vi "robotimageprocessing2.vi"(0 "Image In":T2, 7 "error in":errorcluster) -> (20 "Image Out":T2, 21 "Number of Matches (Shape Matching 1)":i32, 22 "Shape Report (Shape Matching 1)":T1(array[cluster]) {"Score" format="%.2f"; "Centroid"."y" format="%.2f"; "Centroid"."x" format="%.2f"}, 23 "Shape Report (calibrated) (Shape Matching 1)":T1(array[cluster]) {"Score" format="%.2f"; "Centroid"."y" format="%.2f"; "Centroid"."x" format="%.2f"}, 27 "error out":errorcluster)   [LabVIEW 2015]
uses:
  <vilib>/vision/Image Controls.llb/IMAQ Image.ctl
  <vilib>/vision/NI_Vision_Development_Module.lvlib
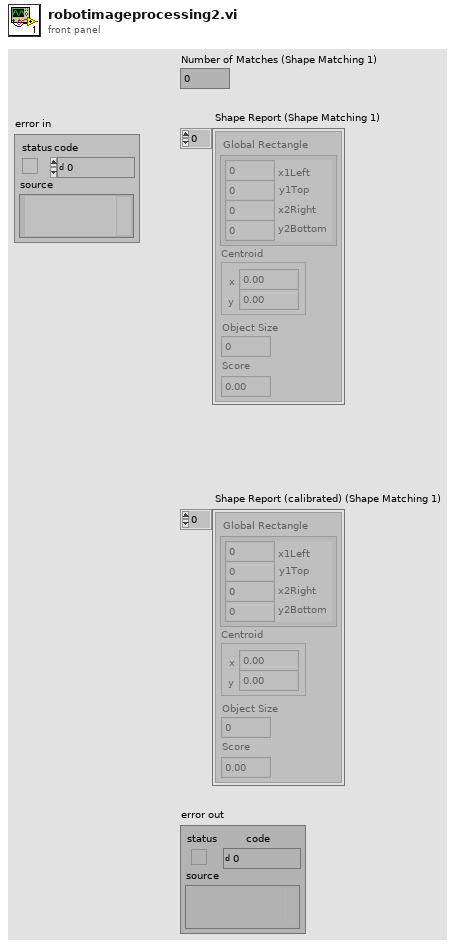
[diagram p1: front panel]
types:
  T1 = cluster{"Global Rectangle":cluster{"x1Left":i32, "y1Top":i32, "x2Right":i32, "y2Bottom":i32}, "Centroid":cluster{"x":sgl, "y":sgl}, "Object Size":u32, "Score":dbl}[]
  T2 = typedef "IMAQ Image.ctl" = refnum<image>
  T3 = enum32{"AutoM", "Close", "Dilate", "Erode", "Gradient", "Gradient out", "Gradient in", "Hit miss", "Open", "PClose", "POpen", "Thick", "Thin"}
  T4 = cluster{"Measurement Parameter":i32, "Range Lower Value":dbl, "Range Upper Value":dbl, "Range":bool, "Measurement Type":bool}[]
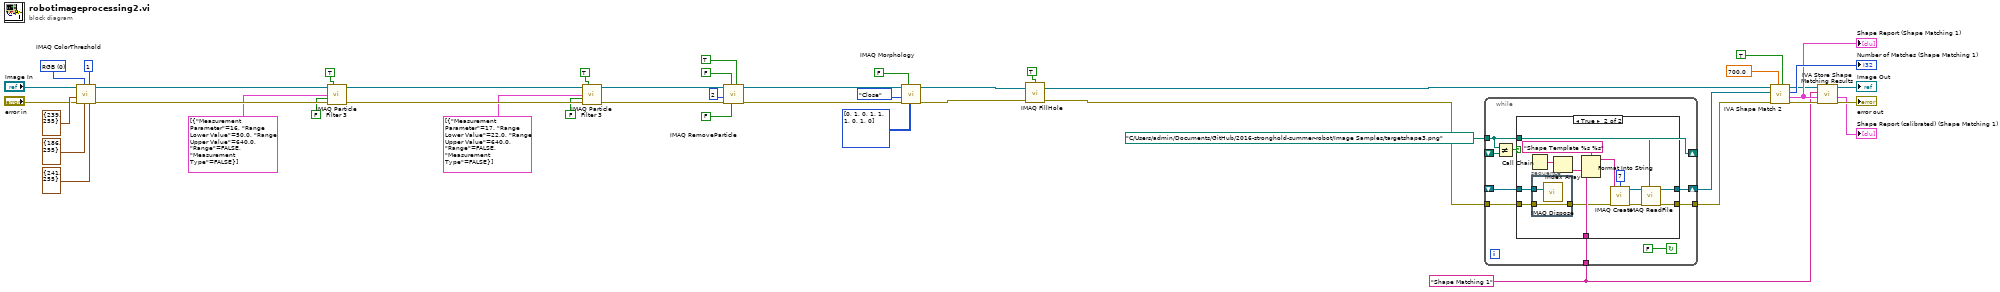
[diagram p0: block diagram]
diagram:
  w1 = "Shape Matching 1" ("Step Name")
  w45 = u16 0 items=["RGB", "HSL", "HSV", "HSI"] ("Color Mode")
  n1 = call "IMAQ ColorThreshold"("Blue or Luma or Val or Inten Range"=cluster{"Lower value":i32, "Upper value":i32} {"Lower value"=241, "Upper value"=255}, "Replace Value"=1, "Green or Sat Range"=cluster{"Lower value":i32, "Upper value":i32} {"Lower value"=186, "Upper value"=255}, "Color Mode"=w45, "error in (no error)"="error in", "Red or Hue Range"=cluster{"Lower value":i32, "Upper value":i32} {"Lower value"=239, "Upper value"=255}, "Image Src"="Image In") -> ("error out"=w39:errorcluster, "Image Dst Out"=w35:T2)  [unwired: 1 in, 2 out]
  n2 = call "IMAQ Particle Filter 3"("Image Src"=w35, "Connectivity 4/8 (8)"=TRUE, "Selection Values"=T4 [{"Measurement Parameter"=16, "Range Lower Value"=50.0, "Range Upper Value"=640.0, "Range"=FALSE, "Measurement Type"=FALSE}], "Keep/Remove Particles (F)"=FALSE ("Keep/Remove Particles"), "error in (no error)"=w39) -> ("Image Dst Out"=w30:T2, "error out"=w36:errorcluster)  [unwired: 4 in, 5 out]
  n3 = call "IMAQ Particle Filter 3"("Image Src"=w30, "Connectivity 4/8 (8)"=TRUE, "Selection Values"=T4 [{"Measurement Parameter"=17, "Range Lower Value"=22.0, "Range Upper Value"=640.0, "Range"=FALSE, "Measurement Type"=FALSE}], "Keep/Remove Particles (F)"=FALSE ("Keep/Remove Particles"), "error in (no error)"=w36) -> ("Image Dst Out"=w24:T2, "error out"=w31:errorcluster)  [unwired: 4 in, 5 out]
  n4 = call "IMAQ RemoveParticle"("Connectivity 4/8 (8)"=TRUE, "Low Pass/High Pass (Low)"=FALSE, "Square/Hexa (Square)"=FALSE, "error in (no error)"=w31, "Number of Erosion"=2, "Image Src"=w24) -> ("error out"=w23:errorcluster, "Image Dst Out"=w19:T2)  [unwired: 1 in, 3 out]
  n5 = call "IMAQ Morphology"("Structuring Element"=i32[][] [[0, 1, 0], [1, 1, 1], [0, 1, 0]], "Square/Hexa (Square)"=FALSE, "error in (no error)"=w23, "Operation"=T3."Close", "Image Src"=w19) -> ("error out"=w18:errorcluster, "Image Dst Out"=w16:T2)  [unwired: 2 in, 3 out]
  n6 = call "IMAQ FillHole"("error in (no error)"=w18, "Image Src"=w16, "Connectivity 4/8 (8)"=TRUE) -> ("error out"=w15:errorcluster, "Image Dst Out"=w11:T2)  [unwired: 1 in, 2 out]
  n7 = while {
    shift-right: [w55] -> w2
    shift-left: _ -> [w54]
    tunnel: [w52] -> w3
    tunnel: w15 -> [w51]
    tunnel: path "C:/Users/admin/Documents/GitHub/2016-stronghold-summer-robot/Image Samples/targetshape3.png" ("Template Path") -> [w49]
    tunnel: w1 -> [w50]
    shift-right: [w49] -> _
    shift-left: _ -> [w48]
    stop <- FALSE continue-if-true
    n8 = Not Equal?(x=w49, y=w48) -> (x != y?=w47:bool)
    n9 = case shown="True" w47 {
      tunnel: [w57 w68] -> w55
      tunnel: w54 -> [w57 w61]
      tunnel: [w56 w66] -> w52
      tunnel: w51 -> [w56 w60]
      tunnel: w49 -> [_ w58]
      tunnel: w50 -> [_ w62]
      frame False {
      }
      frame True {
        n10 = Call Chain() -> (call chain=w64:string[])
        n11 = stacked-sequence {
          tunnel: w61 -> [w73]
          tunnel: w60 -> [w72]
          tunnel: [w72] -> w59
          frame #0 {
            n12 = call "IMAQ Dispose"("Image"=w73) -> ()  [unwired: 2 in, 4 out]
          }
        }
        n13 = Index Array(array=w64) -> (element=w63:string)  [unwired: 1 in]
        n14 = Format Into String(format string="Shape Template %s %s" ("Image Name"), w63, w62) -> (resulting string=w71:string)  [unwired: 2 in, 1 out]
        n15 = call "IMAQ Create"("Border Size"=7, "Image Name"=w71, "error in (no error)"=w59) -> ("New Image"=w69:T2, "error out"=w67:errorcluster)  [unwired: 1 in, 1 out]
        n16 = call "IMAQ ReadFile"("File Path"=w58, "error in (no error)"=w67, "Image"=w69) -> ("error out"=w66:errorcluster, "Image Out"=w68:T2)  [unwired: 2 in, 5 out]
      }
    }
  }
  n17 = call <vilib>:"IVA Shape Match 2.vi"("Scale Invariance"=TRUE, "Minimal Score"=700.0, "error in (no error)"=w3, "Template"=w2, "Image Src"=w11) -> ("error out"=w10:errorcluster, "Shape Report"=w8:T1, "Number of Matches"=→"Number of Matches (Shape Matching 1)":i32, "Image Out"=w7:T2)  [unwired: 3 out]
  "Shape Report (Shape Matching 1)" <- w8
  n18 = call <vilib>:"IVA Store Shape Matching Results.vi"("error in (no error)"=w10, "Shape Report"=w8, "Step Name"=w1, "Image in"=w7) -> ("error out"=→"error out":errorcluster, "Shape Report (calibrated)"=→"Shape Report (calibrated) (Shape Matching 1)":T1, "Image dup"=→"Image Out":T2)  [unwired: 5 out]
